vi "Shift Register.vi"() -> ()   [LabVIEW 2018]
panel:
  out "Numeric 4":i32
  out "Numeric 3":i32
  out "Numeric 2":i32
  out "Before":i8
  out "Numeric":i8
  in  "stop":bool
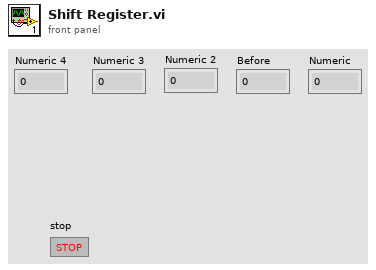
[diagram p1: front panel]
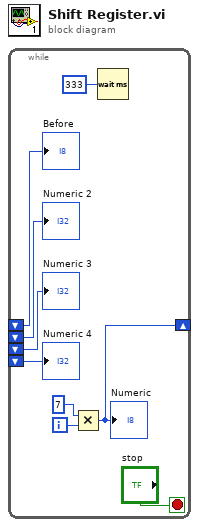
[diagram p0: block diagram]
diagram:
  n1 = while {
    shift-right: [w1] -> _
    shift-left: _ -> [w7]
    shift-left: _ -> [w6]
    shift-left: _ -> [w5]
    shift-left: _ -> [w4]
    i -> [w3]
    stop <- "stop" stop-if-true
    n2 = Multiply(x=7 ("y"), y=w3) -> (x*y=w1:i32)
    "Numeric" <- w1
    n3 = Wait (ms)(milliseconds to wait=u32 333) -> ()  [unwired: 1 out]
    "Before" <- w7
    "Numeric 2" <- w6
    "Numeric 3" <- w5
    "Numeric 4" <- w4
  }
